vi "shooter_hood.vi"(10 "Enable Hood":bool) -> ()   [LabVIEW 2020]
uses:
  <vilib>/Rock Robotics/WPI/ThirdParty/REV Robotics/REVLib/Typedef/Spark MAX Control Type.ctl
  <vilib>/Rock Robotics/WPI/ThirdParty/Phoenix-LabVIEW/Motor Controller/Controls/CTRE_Phoenix_MotorControl_ControlMode.ctl
  Robot Global Data.vi
  TitanLib/Lib/TitanLib.lvlib
panel:
  out "Sensor Position":dbl
  in  "Zero Hood":bool
  in  "Hood Setpoint (deg)":dbl
  in  "CTRE Hood Constants":T1
  in  "Max Velocity":dbl
  in  "REV PID Constants":T2={"P Gain"=0.0, "I Gain"=0.0, "D Gain"=0.0, "F Gain"=0.0, "I Zone"=0.0, "Min Output"=-1.0, "Max Output"=1.0}
  in  "Max Acceleration":dbl
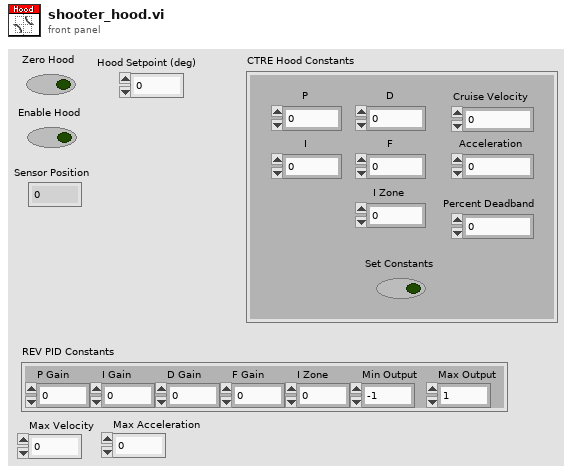
[diagram p1: front panel]
types:
  T1 = cluster{"Set Constants":bool, "P":dbl, "I":dbl, "D":dbl, "F":dbl, "I Zone":dbl, "Cruise Velocity":i32, "Acceleration":i32, "Percent Deadband":dbl}
  T2 = cluster{"P Gain":dbl, "I Gain":dbl, "D Gain":dbl, "F Gain":dbl, "I Zone":dbl, "Min Output":dbl, "Max Output":dbl}
  T3 = typedef "robot.ctl" = enum16{"Hyperion", "Theia"}
  T4 = typedef "Spark MAX Control Type.ctl" = enum16{"Percent VBus", "Voltage", "Velocity", "Position", "Smart Motion", "Current", "Smart Velocity"}
  T5 = typedef "WPI_MotorControlDeviceRef.ctl" = cluster{"DeviceStatus":errorcluster, "Type":T6, "PWM":cluster{"PWM Channel":T7, "DeadBand":T8}, "CAN":cluster{"Device Number":u8, "SetOutput VI Ref":variant, "GetOutput VI Ref":variant, "Enable VI Ref":variant, "Disable VI Ref":variant, "Data":variant}, "Invert":bool, "DIO PWM":cluster{"PWM \"Enable\" Channel":T7, "DIOChannel":T9, "PWM Rate":dbl}}
  T6 = typedef "WPI_MotorControlType.ctl" = enum16{"PWM", "CAN", "DIO PWM"}
  T7 = typedef "FPGA_DIOPWMChannel.ctl" = enum8{"PWM 0", "PWM 1", "PWM 2", "PWM 3", "PWM 4", "PWM 5", "PWM 6", "PWM 7", "PWM 8", "PWM 9", "PWM MXP 0", "PWM MXP 1", "PWM MXP 2", "PWM MXP 3", "PWM MXP 4", "PWM MXP 5", "PWM MXP 6", "PWM MXP 7", "PWM MXP 8", "PWM MXP 9", "Invalid"}
  T8 = typedef "WPI_PWMDeadband.ctl" = cluster{"Name":string, "maxPositivePwm":i32, "minPositivePwm":i32, "centerPwm":i32, "maxNegativePwm":i32, "minNegativePwm":i32, "angularRange":u16}
  T9 = typedef "FPGA_DIOChannel.ctl" = enum8{"DIO 0", "DIO 1", "DIO 2", "DIO 3", "DIO 4", "DIO 5", "DIO 6", "DIO 7", "DIO 8", "DIO 9", "DIO MXP 0", "DIO MXP 1", "DIO MXP 2", "DIO MXP 3", "DIO MXP 4", "DIO MXP 5", "DIO MXP 6", "DIO MXP 7", "DIO MXP 8", "DIO MXP 9", "DIO MXP 10", "DIO MXP 11", "DIO MXP 12", "DIO MXP 13", "DIO MXP 14", "DIO MXP 15", "SPI Port CS1", "SPI Port CS2", "SPI Port CS3", "SPI Port MISO", "SPI Port MOSI", "Invalid"}
  T10 = typedef "CTRE_Phoenix_MotorControl_ControlMode.ctl" = u16
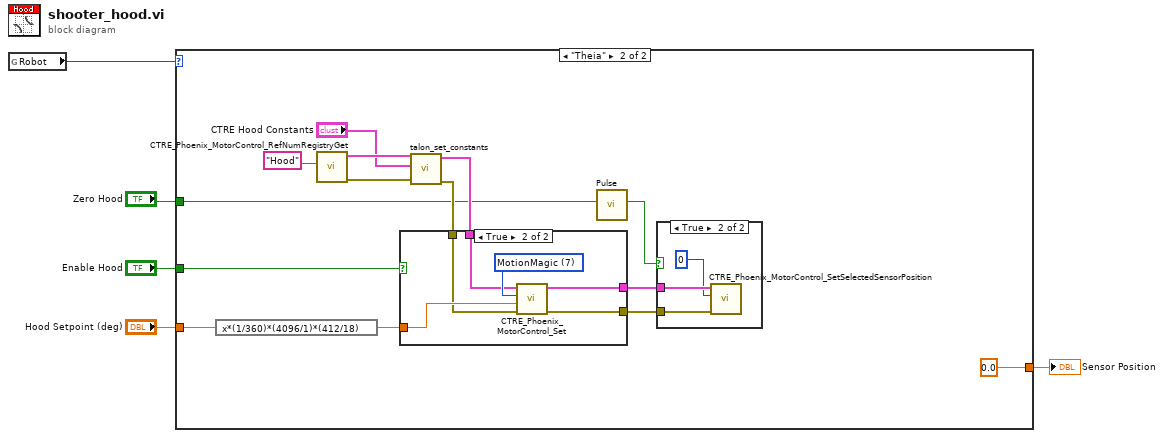
[diagram p0: block diagram]
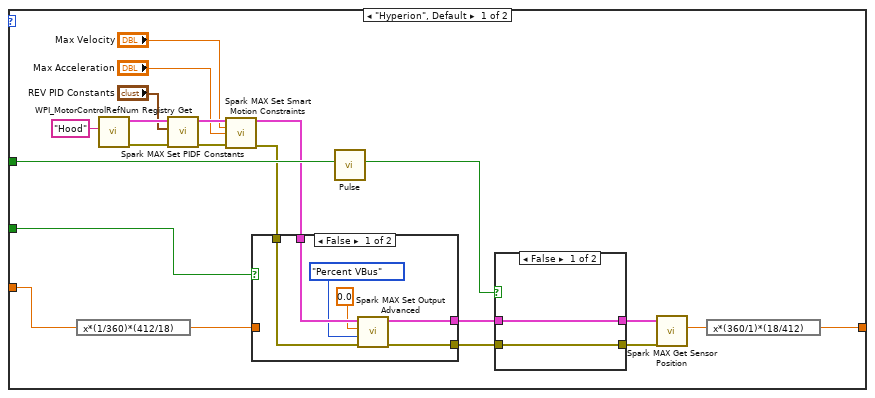
[diagram p2: hidden frame]
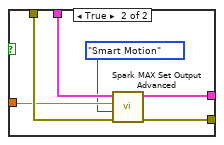
[diagram p3: hidden frame]
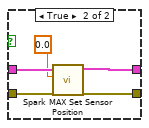
[diagram p4: hidden frame]
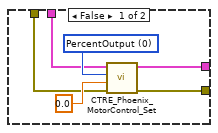
[diagram p5: hidden frame]
diagram:
  n1 = global read "Robot Global Data.vi" "Robot"() -> (w1:T3)
  n2 = case shown="\"Theia\"" w1 {
    tunnel: "Zero Hood" -> [w22 w47]
    tunnel: "Enable Hood" -> [w17 w52]
    tunnel: [w11 0.0 ("Sensor Position")] -> w3
    tunnel: "Hood Setpoint (deg)" -> [w14 w50]
    frame "Hyperion", Default {
      n3 = expression code="x*(1/360)*(412/18)"(w14) -> (w13:dbl)
      n4 = call <vilib>:"WPI_MotorControlRefNum Registry Get.vi"("refnum name"="Hood") -> ("error out"=w25:errorcluster, "MotorControlDevRef"=w24:T5)  [unwired: 9 in]
      n5 = call <vilib>:"Spark MAX Set PIDF Constants.vi"("error in"=w25, "PID Constants"="REV PID Constants", "MotorControlDeviceRef"=w24) -> ("error out"=w9:errorcluster, "MotorControlDeviceRef"=w10:T5)  [unwired: 7 in]
      n6 = call <vilib>:"Spark MAX Set Smart Motion Constraints.vi"("MotorControlDeviceRef"=w10, "Max Velocity"="Max Velocity", "Max Acceleration"="Max Acceleration", "error in"=w9) -> ("MotorControlDeviceRef"=w21:T5, "error out"=w20:errorcluster)  [unwired: 10 in]
      n7 = case shown="False" w17 {
        tunnel: w21 -> [w32 w38]
        tunnel: w20 -> [w31 w37]
        tunnel: [w28 w36] -> w19
        tunnel: [w27 w35] -> w18
        tunnel: w13 -> [_ w34]
        frame False {
          n8 = call <vilib>:"Spark MAX Set Output Advanced.vi"("error in (no error)"=w31, "Control Mode"=Spark_MAX_Control_Type."Percent VBus", "Setpoint"=0.0, "MotorControlDevRef"=w32) -> ("error out"=w27:errorcluster, "MotorControlDevRef"=w28:T5)  [unwired: 6 in]
        }
        frame True {
          n9 = call <vilib>:"Spark MAX Set Output Advanced.vi"("error in (no error)"=w37, "Control Mode"=Spark_MAX_Control_Type."Smart Motion", "Setpoint"=w34, "MotorControlDevRef"=w38) -> ("error out"=w35:errorcluster, "MotorControlDevRef"=w36:T5)  [unwired: 6 in]
        }
      }
      n10 = call "Pulse.vi"("Input"=w22) -> ("Output"=w23:bool)  [unwired: 10 in]
      n11 = case shown="False" w23 {
        tunnel: w19 -> [w40 w45]
        tunnel: w18 -> [w39 w44]
        tunnel: [w40 w42] -> w16
        tunnel: [w39 w41] -> w15
        frame False {
        }
        frame True {
          n12 = call <vilib>:"Spark MAX Set Sensor Position.vi"("error in"=w44, "Position"=0.0, "MotorControlDeviceRef"=w45) -> ("error out"=w41:errorcluster, "MotorControlDeviceRef"=w42:T5)  [unwired: 7 in]
        }
      }
      n13 = call <vilib>:"Spark MAX Get Sensor Position.vi"("error in (no error)"=w15, "MotorControlDevRef in"=w16) -> ("Sensor Position"=w12:dbl)  [unwired: 6 in, 3 out]
      n14 = expression code="x*(360/1)*(18/412)"(w12) -> (w11:dbl)
    }
    frame "Theia" {
      n15 = expression code="x*(1/360)*(4096/1)*(412/18)"(w50) -> (w49:dbl)
      n16 = call <vilib>:"CTRE_Phoenix_MotorControl_RefNumRegistryGet.vi"("refnum name"="Hood") -> ("error out"=w57:errorcluster, "PhoenixMotorControlDevRef"=w58:T5)  [unwired: 9 in]
      n17 = call "talon_set_constants.vi"("error in"=w57, "Constants"="CTRE Hood Constants", "PhoenixMotorControlDevRef"=w58) -> ("error out"=w54:errorcluster, "PhoenixMotorControlDevRef"=w53:T5)  [unwired: 7 in]
      n18 = case shown="True" w52 {
        tunnel: [w61 w70] -> w56
        tunnel: [w60 w69] -> w55
        tunnel: w49 -> [_ w68]
        tunnel: w54 -> [w62 w67]
        tunnel: w53 -> [w63 w66]
        frame False {
          w65 = T10 0 items=["PercentOutput"=0, "Position"=1, "Velocity"=2, "Current"=3, "Follower"=5, "MotionProfile"=6, "MotionMagic"=7, "MotionProfileArc"=10, "Disabled"=15] ("Control Mode")
          n19 = call <vilib>:"CTRE_Phoenix_MotorControl_Set.vi"("error in (no error)"=w62, "Output"=0.0, "Control Mode"=w65, "PhoenixMotorControlDevRef"=w63) -> ("error out"=w60:errorcluster, "PhoenixMotorControlDevRef"=w61:T5)  [unwired: 6 in]
        }
        frame True {
          w71 = T10 7 items=["PercentOutput"=0, "Position"=1, "Velocity"=2, "Current"=3, "Follower"=5, "MotionProfile"=6, "MotionMagic"=7, "MotionProfileArc"=10, "Disabled"=15] ("Control Mode")
          n20 = call <vilib>:"CTRE_Phoenix_MotorControl_Set.vi"("error in (no error)"=w67, "Output"=w68, "Control Mode"=w71, "PhoenixMotorControlDevRef"=w66) -> ("error out"=w69:errorcluster, "PhoenixMotorControlDevRef"=w70:T5)  [unwired: 6 in]
        }
      }
      n21 = call "Pulse.vi"("Input"=w47) -> ("Output"=w46:bool)  [unwired: 10 in]
      n22 = case shown="True" w46 {
        tunnel: w56 -> [_ w74]
        tunnel: w55 -> [_ w73]
        frame False {
        }
        frame True {
          n23 = call <vilib>:"CTRE_Phoenix_MotorControl_SetSelectedSensorPosition.vi"("error in (no error)"=w73, "New Sensor Position"=0, "PhoenixMotorControlDevRef"=w74) -> ()  [unwired: 7 in, 2 out]
        }
      }
    }
  }
  "Sensor Position" <- w3
